vi "Circumference of circle.vi"() -> ()   [LabVIEW 2020]
panel:
  out "Circumference":dbl format="%#_4g"
  in  "Radius":dbl(knob) scale=0.0..10.0
  # "Circumference of circle"
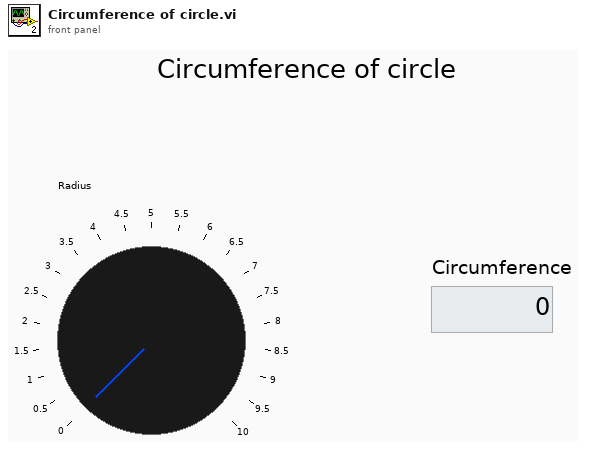
[diagram p1: front panel]
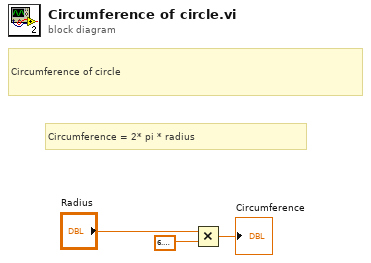
[diagram p0: block diagram]
diagram:
  # "Circumference = 2* pi * radius"
  # "Circumference of circle"
  n1 = Multiply(x="Radius", y=6.283185307179586) -> (x*y=→"Circumference":dbl)
